vi "Delete Temporary Template Directory.vi"(11 "Target Template Root Dir":path) -> ()   [LabVIEW 2013]
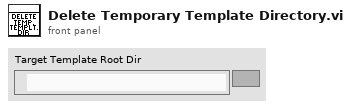
[diagram p1: front panel]
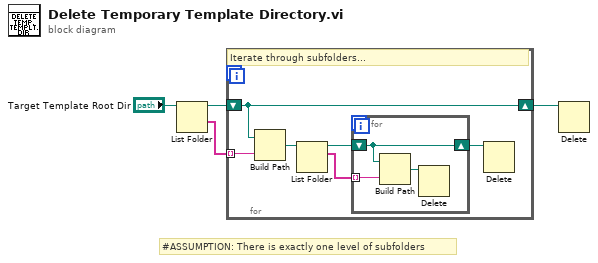
[diagram p0: block diagram]
diagram:
  # "#ASSUMPTION: There is exactly one level of subfolders"
  n1 = List Folder(path="Target Template Root Dir") -> (path out=w3:path, folder names=w1:string[])  [unwired: 3 in, 2 out]
  n2 = for {
    tunnel: w1 -> [w10] mode=indexing
    shift-right: [w9] -> w2
    shift-left: w3 -> [w9]
    # "Iterate through subfolders..."
    n3 = Build Path(base path=w9, name or relative path=w10) -> (appended path=w8:path)
    n4 = List Folder(path=w8) -> (path out=w7:path, filenames=w6:string[])  [unwired: 3 in, 2 out]
    n5 = for {
      tunnel: w6 -> [w12] mode=indexing
      shift-right: [w11] -> w5
      shift-left: w7 -> [w11]
      n6 = Build Path(base path=w11, name or relative path=w12) -> (appended path=w13:path)
      n7 = Delete(path (use dialog)=w13) -> ()  [unwired: 4 in, 3 out]
    }
    n8 = Delete(path (use dialog)=w5) -> ()  [unwired: 4 in, 3 out]
  }
  n9 = Delete(path (use dialog)=w2) -> ()  [unwired: 4 in, 3 out]
